vi "NT_LL_Write Boolean Array.vi"(8 "error in (no error)":errorcluster, 9 "value":bool[](array[boolean]), 10 "timestamp":u64, 11 "publishHandle":u32) -> (0 "error out":errorcluster, 3 "success":u32)   [LabVIEW 2025]
uses:
  ntcoreffi.dll
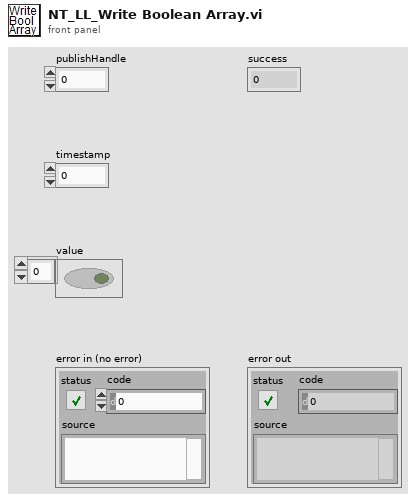
[diagram p1: front panel]
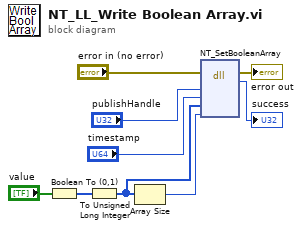
[diagram p0: block diagram]
diagram:
  n1 = Boolean To (0,1)(Boolean="value") -> (0, 1=w7:i16[])
  n2 = To Unsigned Long Integer(number=w7) -> (unsigned 32bit integer=w9:u32[])
  n3 = Array Size(array=w9) -> (size(s)=w8:i32)
  n4 = dll-call lib="ntcoreffi.*" fn="NT_SetBooleanArray"(error in="error in (no error)", "publishHandle"="publishHandle", "time"="timestamp", "value"=w9, "arraySz"=w8) -> (error out=→"error out":errorcluster, "success"=→"success":u32)  [unwired: 6 in, 1 out]
